vi "DuplicateCells.vi"(6 "# Rows":i32, 8 "error in (no error)":errorcluster, 9 "Table CtlRef In":refnum<vi>, 10 "Cell Position":T1, 11 "Column in":refnum<class "Column.lvclass">) -> (0 "error out":errorcluster, 1 "Table CtlRef Out":refnum<vi>, 3 "Column out":refnum<class "Column.lvclass">)   [LabVIEW 2013, in "Column.lvclass"]
doc: "Intended to be used as part of Insert Row(s) function, this method only copies formatting. Values can be more efficiently duplicated by row with array functions.\n\nThe funcitonality was made column-specific so that SingleVal can be handled appropriately."
uses:
  Column.lvclass
  <vilib>/Utility/miscctls.llb/LVRowAndColumnTypeDef.ctl
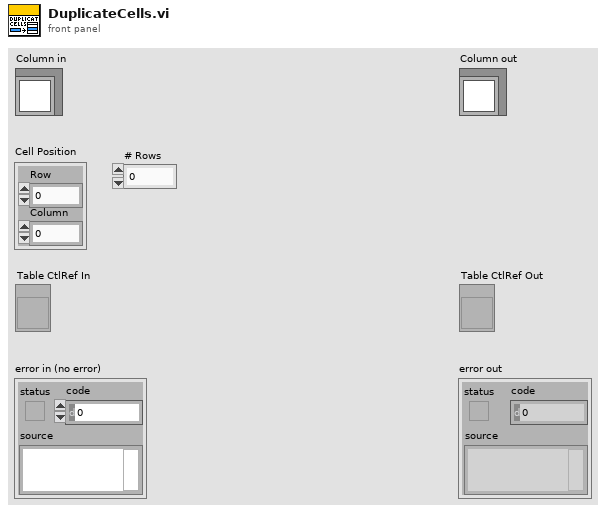
[diagram p1: front panel]
types:
  T1 = typedef "LVRowAndColumnTypeDef.ctl" = cluster{"Row":i32, "Column":i32}
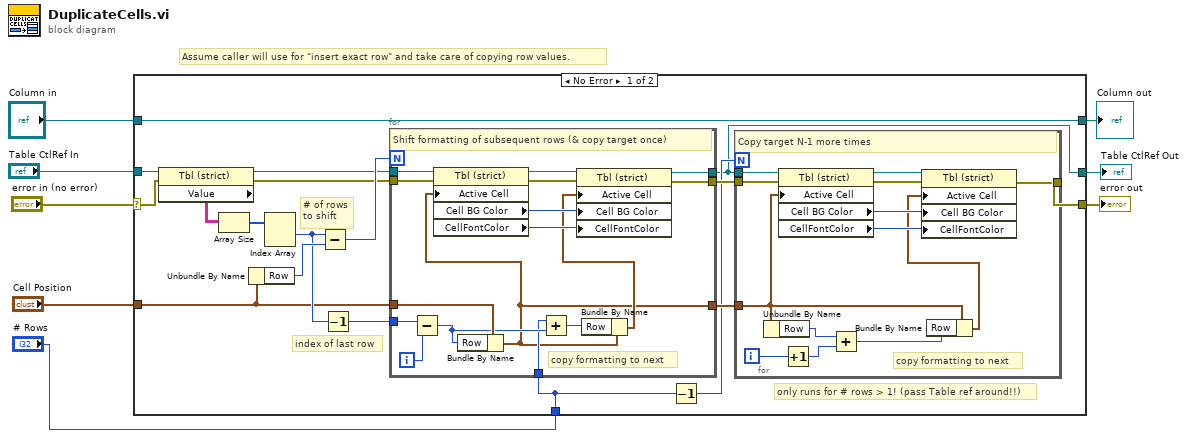
[diagram p0: block diagram]
diagram:
  # "Assume caller will use for \"insert exact row\" and take care of copying row values."
  n1 = case shown="No Error" "error in (no error)" {
    selector: "error in (no error)" -> [w21 w58]
    tunnel: [w14 w58] -> w7
    tunnel: [w26 w57] -> w5
    tunnel: "Column in" -> [w26 w57]
    tunnel: "Table CtlRef In" -> [w25 w56]
    tunnel: [w9 w56] -> w3
    tunnel: "Cell Position" -> [w15 _]
    tunnel: "# Rows" -> [w11 _]
    frame No Error {
      # "only runs for # rows > 1! (pass Table ref around!!)"
      # "index of last row"
      # "# of rows\nto shift"
      n2 = property class="Tbl (strict)"(reference=w25, error in=w21) -> (reference out=w19:refnum<vi>, error out=w18:errorcluster, "Value"=w24:string[][])
      n3 = Array Size(array=w24) -> (size(s)=w23:i32[])
      n4 = Unbundle By Name(w15) -> ("Row"=w22:i32)
      n5 = Index Array(array=w23) -> (element #1=w17:i32)  [unwired: 2 in, 1 out]
      n6 = Subtract(x=w17, y=w22) -> (x-y=w20:i32)
      n7 = Decrement(x=w17) -> (x-1=w16:i32)
      n8 = for {
        N: w20 -> [_]
        tunnel: w19 -> [w52]
        tunnel: w18 -> [w51]
        tunnel: w16 -> [w55]
        tunnel: w15 -> [w53]
        tunnel: [w48] -> w9
        tunnel: [w47] -> w13
        tunnel: w11 -> [w41]
        tunnel: [w40] -> w12
        i -> [w54]
        # "copy formatting to next"
        # "Shift formatting of subsequent rows (& copy target once)"
        n9 = Subtract(x=w55, y=w54) -> (x-y=w44:i32)
        n10 = Bundle By Name(cluster=w53, "Row"=w44) -> (w40:T1)
        n11 = property class="Tbl (strict)"(reference=w52, error in=w51, "Active Cell"=w40) -> (reference out=w50:refnum<vi>, error out=w49:errorcluster, "Cell BG Color"=w46:u32, "CellFontColor"=w45:u32)
        n12 = Add(x=w41, y=w44) -> (x+y=w43:i32)
        n13 = Bundle By Name(cluster=w40, "Row"=w43) -> (w42:T1)
        n14 = property class="Tbl (strict)"(reference=w50, error in=w49, "Active Cell"=w42, "Cell BG Color"=w46, "CellFontColor"=w45) -> (reference out=w48:refnum<vi>, error out=w47:errorcluster)
      }
      n15 = Decrement(x=w11) -> (x-1=w10:i32)
      n16 = for {
        N: w10 -> [_]
        tunnel: w9 -> [w39]
        tunnel: w13 -> [w38]
        tunnel: w12 -> [w29]
        tunnel: [w35] -> w14
        i -> [w28]
        # "copy formatting to next"
        # "Copy target N-1 more times"
        n17 = Unbundle By Name(w29) -> ("Row"=w30:i32)
        n18 = property class="Tbl (strict)"(reference=w39, error in=w38, "Active Cell"=w29) -> (reference out=w37:refnum<vi>, error out=w36:errorcluster, "Cell BG Color"=w34:u32, "CellFontColor"=w33:u32)
        n19 = Increment(x=w28) -> (x+1=w27:i32)
        n20 = Add(x=w30, y=w27) -> (x+y=w32:i32)
        n21 = Bundle By Name(cluster=w29, "Row"=w32) -> (w31:T1)
        n22 = property class="Tbl (strict)"(reference=w37, error in=w36, "Active Cell"=w31, "Cell BG Color"=w34, "CellFontColor"=w33) -> (error out=w35:errorcluster)  [unwired: 1 out]
      }
    }
    frame Error {
    }
  }
  "error out" <- w7
  "Column out" <- w5
  "Table CtlRef Out" <- w3
